vi "Identify Pin Types.vi"(0 "TSM context":T2, 5 "Pins and/or Pin Groups":tag[](array[tag]), 11 "error in":errorcluster) -> (4 "Pin Types":T1[](array[typedef]), 8 "Pin Group Found?":bool, 15 "error out":errorcluster)   [LabVIEW 2019]
uses:
  <vilib>/NI_TestStand_SemiconductorModule/NI_TestStand_Semiconductor_Module.lvlibp/PinMap/General/SemiconductorModuleContext.ctl
  TSM Pin Type Identifier.ctl
  <vilib>/NI_TestStand_SemiconductorModule/NI_TestStand_Semiconductor_Module.lvlibp
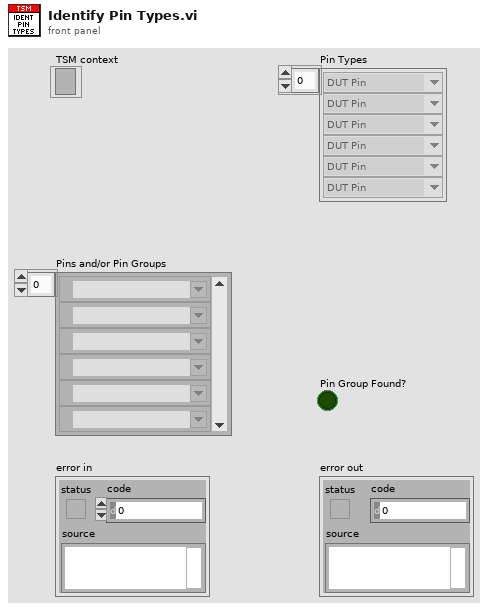
[diagram p1: front panel]
types:
  T1 = typedef "TSM Pin Type Identifier.ctl" = enum8{"DUT Pin", "System Pin", "Pin Group", "Not Determined"}
  T2 = typedef "NI_TestStand_Semiconductor_Module.lvlibp/SemiconductorModuleContext.ctl" = refnum<k7>
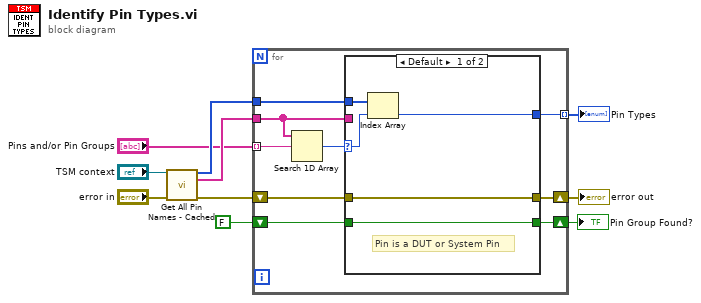
[diagram p0: block diagram]
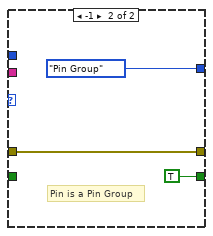
[diagram p2: hidden frame]
diagram:
  n1 = call "Get All Pin Names - Cached.vi"("TSM Context in"="TSM context", "error in"="error in") -> ("Pin Types"=w6:T1[], "Pin Names"=w5:tag[], "error out"=w8:errorcluster)  [unwired: 11 in]
  n2 = for {
    shift-right: [w19] -> w10
    shift-left: w8 -> [w18]
    tunnel: "Pins and/or Pin Groups" -> [w15] mode=indexing
    tunnel: [w16] -> w3 mode=indexing
    tunnel: w6 -> [w14]
    tunnel: w5 -> [w13]
    shift-right: [w11] -> w1
    shift-left: FALSE -> [w12]
    n3 = Search 1D Array(1D array=w13, element=w15) -> (index of element=w17:i32)  [unwired: 1 in]
    n4 = case shown="Default" w17 {
      selector: w17 -> [w22 _]
      tunnel: [w24 w26] -> w19
      tunnel: w18 -> [w24 w26]
      tunnel: w14 -> [w23 _]
      tunnel: [w21 TSM_Pin_Type_Identifier."Pin Group" ("Enum")] -> w16
      tunnel: w13 -> [_ _]
      tunnel: w12 -> [w20 _]
      tunnel: [w20 TRUE] -> w11
      frame Default {
        # "Pin is a DUT or System Pin"
        n5 = Index Array(array=w23, index=w22) -> (element=w21:T1)
      }
      frame -1 {
        # "Pin is a Pin Group"
      }
    }
  }
  "error out" <- w10
  "Pin Types" <- w3
  "Pin Group Found?" <- w1
